vi "Practica_3.vi"() -> ()   [LabVIEW 2020]
panel:
  out "Numeric":dbl
  out "Boolean 2":bool
  in  "LIMITE SUPERIOR":dbl
  in  "Stop Button":bool
  in  "LIMITE INFERIOR":dbl
  # "CONSTRUCCIÓN DE INSTRUMENTOS VIRTUALES PARA EL CONTROL DE VARIABLES FÍSICAS"
  # "TEMPERATURA REGISTRADA"
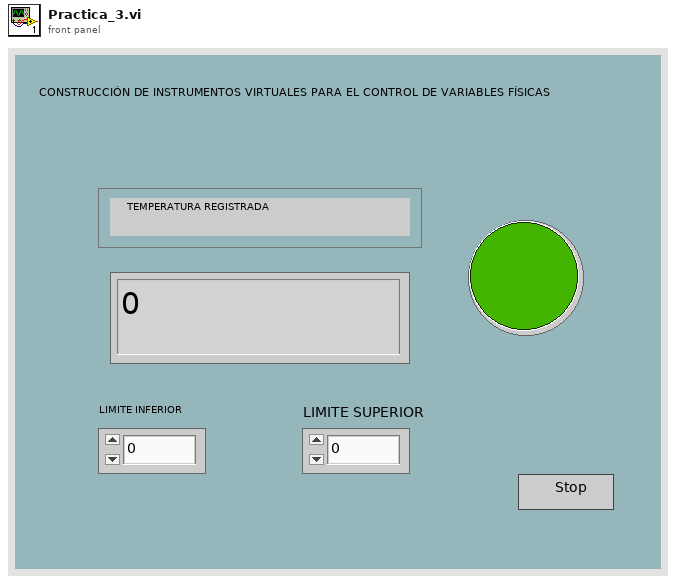
[diagram p1: front panel]
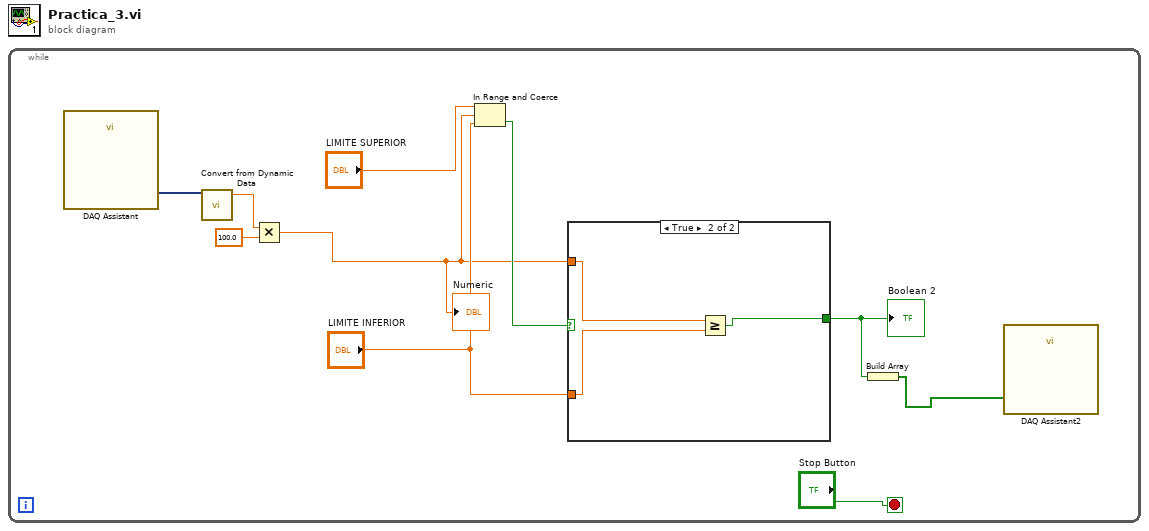
[diagram p0: block diagram]
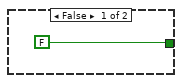
[diagram p2: hidden frame]
diagram:
  n1 = while {
    stop <- "Stop Button" stop-if-true
    n2 = call "DAQ Assistant"() -> ("data"=w5:dynamicdata)  [unwired: 16 in, 3 out]
    n3 = call "Convert from Dynamic Data"("Dynamic Data Type"=w5) -> ("Scalar"=w4:dbl)  [unwired: 3 in]
    n4 = Multiply(x=w4, y=100.0) -> (x*y=w2:dbl)
    "Numeric" <- w2
    n5 = In Range and Coerce(upper limit="LIMITE SUPERIOR", x=w2, lower limit="LIMITE INFERIOR") -> (In Range?=w10:bool)  [unwired: 1 out]
    n6 = case shown="True" w10 {
      tunnel: w2 -> [_ w13]
      tunnel: "LIMITE INFERIOR" -> [_ w14]
      tunnel: [FALSE w12] -> w3
      frame False {
      }
      frame True {
        n7 = Greater Or Equal?(x=w13, y=w14) -> (x >= y?=w12:bool)
      }
    }
    "Boolean 2" <- w3
    n8 = Build Array(w3) -> (w1:bool[])
    n9 = call "DAQ Assistant2"("data"=w1) -> ()  [unwired: 17 in, 2 out]
  }
